vi "曲线处理.vi"(0 "上限":sgl, 1 "下限":sgl, 2 "起点":dbl, 3 "终点":dbl, 4 "历史数据":sgl[](array[numeric])) -> (5 "值":sgl, 6 "示值":string, 7 "曲线数组":sgl[](array[numeric]), 10 "范围内?":bool)   [LabVIEW 2018]
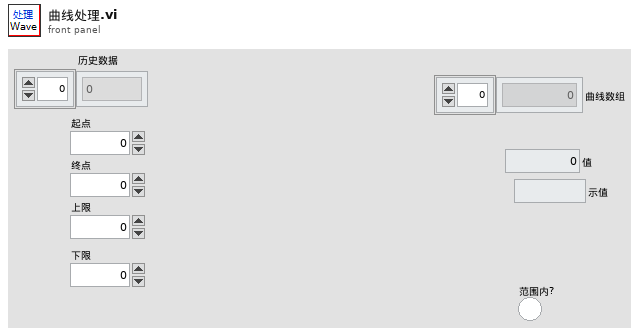
[diagram p1: front panel]
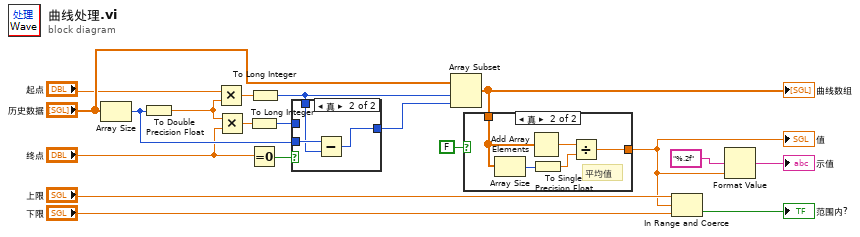
[diagram p0: block diagram]
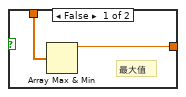
[diagram p2: hidden frame]
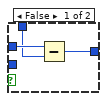
[diagram p3: hidden frame]
diagram:
  n1 = Array Size(array="历史数据") -> (size(s)=w15:i32)
  n2 = To Double Precision Float(number=w15) -> (double precision float=w10:dbl)
  n3 = Multiply(x="起点", y=w10) -> (x*y=w17:dbl)
  n4 = Multiply(x=w10, y="终点") -> (x*y=w16:dbl)
  n5 = To Long Integer(number=w16) -> (32bit integer=w13:i32)
  n6 = Equal To 0?(x="终点") -> (x = 0?=w19:bool)
  n7 = To Long Integer(number=w17) -> (32bit integer=w12:i32)
  n8 = case shown="真" w19 {
    tunnel: w15 -> [_ w25]
    tunnel: w13 -> [w22 _]
    tunnel: w12 -> [w21 w24]
    tunnel: [w20 w23] -> w11
    frame False {
      n9 = Subtract(x=w22, y=w21) -> (x-y=w20:i32)
    }
    frame True {
      n10 = Subtract(x=w25, y=w24) -> (x-y=w23:i32)
    }
  }
  n11 = Array Subset(array="历史数据", index=w12, length=w11) -> (w18:sgl[])
  "曲线数组" <- w18
  n12 = case shown="真" FALSE {
    tunnel: w18 -> [w27 w32]
    tunnel: [w26 w28] -> w3
    frame False {
      # "最大值"
      n13 = Array Max & Min(array=w27) -> (max value=w26:sgl)  [unwired: 3 out]
    }
    frame True {
      # "平均值"
      n14 = Array Size(array=w32) -> (size(s)=w30:i32)
      n15 = Add Array Elements(numeric array=w32) -> (sum=w31:sgl)
      n16 = To Single Precision Float(number=w30) -> (single precision float=w29:sgl)
      n17 = Divide(x=w31, y=w29) -> (x/y=w28:sgl)
    }
  }
  "值" <- w3
  n18 = In Range and Coerce(upper limit="上限", x=w3, lower limit="下限") -> (In Range?=→"范围内?":bool)  [unwired: 1 out]
  n19 = Format Value(format string="%.2f" ("格式字符串"), value (0)=w3) -> (output string=→"示值":string)  [unwired: 1 in]
